vi "RemoveByType.vi"(7 "LabVIEW Object Type":refnum<class>, 8 "error in (no error)":errorcluster, 11 "Collection in":refnum<class "CollectionByValue.lvclass">) -> (0 "error out":errorcluster, 1 "Found":bool, 2 "Removed Objects":refnum<class>[](array[class]), 3 "Collection out":refnum<class "CollectionByValue.lvclass">, 4 "Removed Names":string[](array[string]))   [LabVIEW 2021, in "Collection.lvlib" / "CollectionByValue.lvclass"]
uses:
  CollectionByValue.lvclass
  CollectionByValue.lvclass/CollectionByValue.ctl
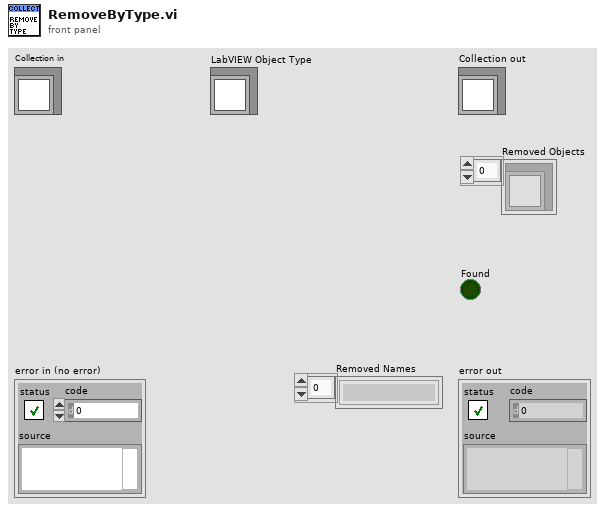
[diagram p1: front panel]
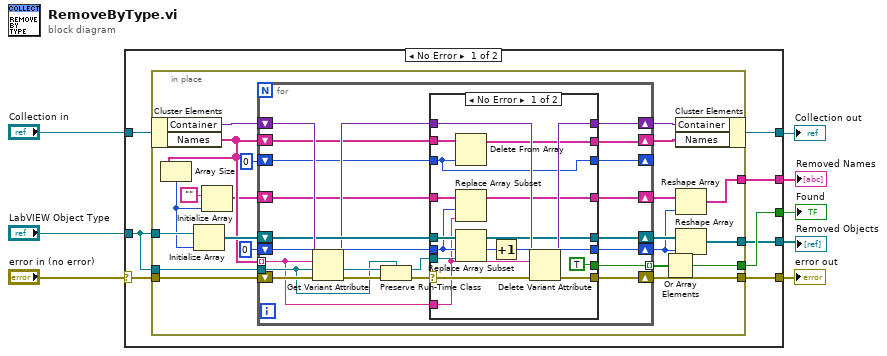
[diagram p0: block diagram]
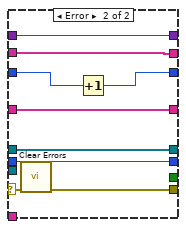
[diagram p2: hidden frame]
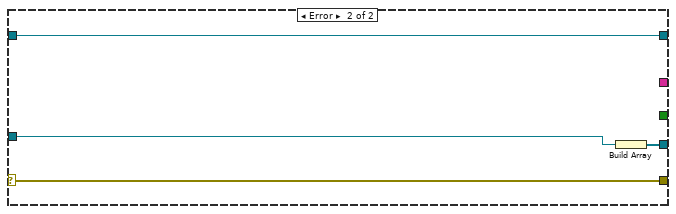
[diagram p3: hidden frame]
diagram:
  n1 = case shown="No Error" "error in (no error)" {
    selector: "error in (no error)" -> [w14 w88]
    tunnel: [w13 w88] -> w5
    tunnel: [w15 w87] -> w7
    tunnel: "Collection in" -> [w16 w87]
    tunnel: "LabVIEW Object Type" -> [w11 w86]
    tunnel: [w12 _] -> w3
    tunnel: [w10 w85] -> w2
    tunnel: [w9 _] -> w1
    frame No Error {
      n2 = in-place {
        in-place-border: w14 -> [w37]
        in-place-border: w11 -> [w33]
        in-place-border: [w34] -> w13
        in-place-border: [w26] -> w12
        in-place-border: w11 -> [w32]
        in-place-border: [w28] -> w10
        in-place-border: [w18] -> w9
        n3 = in-place-cluster #1(w16) -> ("Container"=w36:variant, "Names"=w25:string[])
        n4 = Array Size(array=w25) -> (size(s)=w23:i32)
        n5 = Initialize Array(w32, w23) -> (w31:refnum<class>[])
        n6 = Initialize Array("", w23) -> (w21:string[])
        n7 = for {
          tunnel: w25 -> [w46] mode=indexing
          tunnel: w33 -> [w50]
          shift-right: [w48] -> w34
          shift-left: w37 -> [w59]
          shift-right: [w44] -> w35
          shift-left: w36 -> [w58]
          shift-right: [w53] -> w29
          shift-left: w31 -> [w55]
          shift-right: [w49] -> w20
          shift-left: 0 -> [w54]
          tunnel: [w47] -> w27 mode=indexing
          shift-right: [w42] -> w24
          shift-left: w25 -> [w43]
          shift-right: [w40] -> w19
          shift-left: w21 -> [w41]
          shift-right: [w38] -> _
          shift-left: 0 -> [w39]
          n8 = Get Variant Attribute(Variant=w58, name=w46, default value (empty Variant)=w50, error in=w59) -> (duplicate Variant=w45:variant, value=w51:refnum<class>, error out=w52:errorcluster)  [unwired: 1 out]
          n9 = Preserve Run-Time Class(object in=w51, error in=w52, 2:w50) -> (object out=w56:refnum<class>, error out=w57:errorcluster)
          n10 = case shown="No Error" w57 {
            selector: w57 -> [w73 w82]
            tunnel: w56 -> [w74 _]
            tunnel: w55 -> [w75 w84]
            tunnel: w54 -> [w62 w83]
            tunnel: [w65 w84] -> w53
            tunnel: [w72 w83] -> w49
            tunnel: [w70 w81] -> w48
            tunnel: [TRUE _] -> w47
            tunnel: w46 -> [w61 _]
            tunnel: w45 -> [w69 w80]
            tunnel: [w68 w80] -> w44
            tunnel: w43 -> [w67 w79]
            tunnel: [w66 w79] -> w42
            tunnel: w41 -> [w64 w78]
            tunnel: [w63 w78] -> w40
            tunnel: w39 -> [w60 w77]
            tunnel: [w60 w76] -> w38
            frame No Error {
              n11 = Delete From Array(array=w67, index=w60) -> (array with subset deleted=w66:string[])  [unwired: 1 in, 1 out]
              n12 = Replace Array Subset(array=w64, new element=w61, index=w62) -> (w63:string[])
              n13 = Replace Array Subset(array=w75, new element=w74, index=w62) -> (w65:refnum<class>[])
              n14 = Increment(x=w62) -> (x+1=w72:i32)
              n15 = Delete Variant Attribute(4:w73, 6:w61, 7:w69) -> (0:w70:errorcluster, 3:w68:variant)  [unwired: 1 out]
            }
            frame Error {
              n16 = call <vilib>:"Clear Errors.vi"("error in (no error)"=w82) -> ("error out"=w81:errorcluster)  [unwired: 5 in, 1 out]
              n17 = Increment(x=w77) -> (x+1=w76:i32)
            }
          }
        }
        n18 = Or Array Elements(Boolean array=w27) -> (logical OR=w26:bool)
        n19 = in-place-cluster #1("Container"=w35, "Names"=w24) -> (w15:refnum<class "CollectionByValue.lvclass">)
        n20 = Reshape Array(w19, w20) -> (w18:string[])
        n21 = Reshape Array(w29, w20) -> (w28:refnum<class>[])
      }
    }
    frame Error {
      n22 = Build Array(w86) -> (w85:refnum<class>[])
    }
  }
  "error out" <- w5
  "Collection out" <- w7
  "Found" <- w3
  "Removed Objects" <- w2
  "Removed Names" <- w1
